vi "Teleop.vi"(10 "Match Info":T1={"Autonomous Elapsed Seconds"=0.0, "TeleOp Elapsed Seconds"=0.0, "Disabled Elapsed Seconds"=0.0, "Visited Autonomous"=FALSE, "Visited TeleOp"=FALSE, "Visited Disabled"=FALSE, "Autonomous Settings"={"Autonomous Style"=enum."Independent", "VI Refnum"=refnum}}, 11 "Call Context":T2) -> ()   [LabVIEW 2019]
doc: "This VI is called for each TeleOp packet received from the DS where the robot is not disabled. It is often used to read from the joysticks and update I/O or to update setpoints for timed control loops. It should complete and return within 20 milliseconds or it may miss DS packets."
uses:
  <vilib>/Rock Robotics/Network Tables/NT Read Boolean.vi
  572ad318-ad2d-41da-8177-273dc494c89e.vi
  <vilib>/Rock Robotics/WPI/ThirdParty/Phoenix-LabVIEW/Motor Controller/Controls/CTRE_Phoenix_MotorControl_ControlMode.ctl
  <vilib>/Rock Robotics/WPI/ThirdParty/Phoenix-LabVIEW/Motor Controller/Controls/CTRE_Phoenix_MotorControl_MotionProfileControlMode.ctl
  <vilib>/Rock Robotics/Network Tables/NT Write Numeric Array.vi
  <vilib>/Rock Robotics/Network Tables/NT Read Number.vi
  <vilib>/Rock Robotics/WPI/DriverStation/WPI_DriverStationDerivedRobotMode.ctl
  <vilib>/Rock Robotics/WPI/DriverStation/WPI_DriverStationMatch Info.ctl
panel:
  out "Btm Mot Prof Count 4":i32
  out "Top Mot Prof Count 4":i32
  out "Mot Prof Active Is Valid 4":bool
  out "Mot Prof Active Is Last 4":bool
  out "Mot Prof  Has Under Run 4":bool
  out "Mot Prof  Is Under Run 4":bool
  out "Mot Prof Active Position 4":dbl
  out "Mot Prof Active Velocity 4":dbl
  out "Btm Mot Prof Count 3":i32
  out "Top Mot Prof Count 3":i32
  out "Mot Prof Active Is Valid 3":bool
  out "Mot Prof Active Is Last 3":bool
  out "Mot Prof  Has Under Run 3":bool
  out "Mot Prof  Is Under Run 3":bool
  out "Mot Prof Active Position 3":dbl
  out "Mot Prof Active Velocity 3":dbl
  out "Btm Mot Prof Count 2":i32
  out "Top Mot Prof Count 2":i32
  out "Mot Prof Active Is Valid 2":bool
  out "Mot Prof Active Is Last 2":bool
  out "Mot Prof  Has Under Run 2":bool
  out "Mot Prof  Is Under Run 2":bool
  out "Mot Prof Active Position 2":dbl
  out "Mot Prof Active Velocity 2":dbl
  out "Is Motion Profile Finished?":bool
  out "Btm Mot Prof Count":i32
  out "Top Mot Prof Count":i32
  out "Mot Prof Active Is Valid":bool
  out "Mot Prof Active Is Last":bool
  out "Mot Prof  Has Under Run":bool
  out "Mot Prof  Is Under Run":bool
  out "Mot Prof Active Position":dbl
  out "Mot Prof Active Velocity":dbl
  out "Sample Slider 0":dbl(slide) scale=0.0..5.0
  out "Sample Boolean 1":bool
  out "Sample Boolean 0":bool
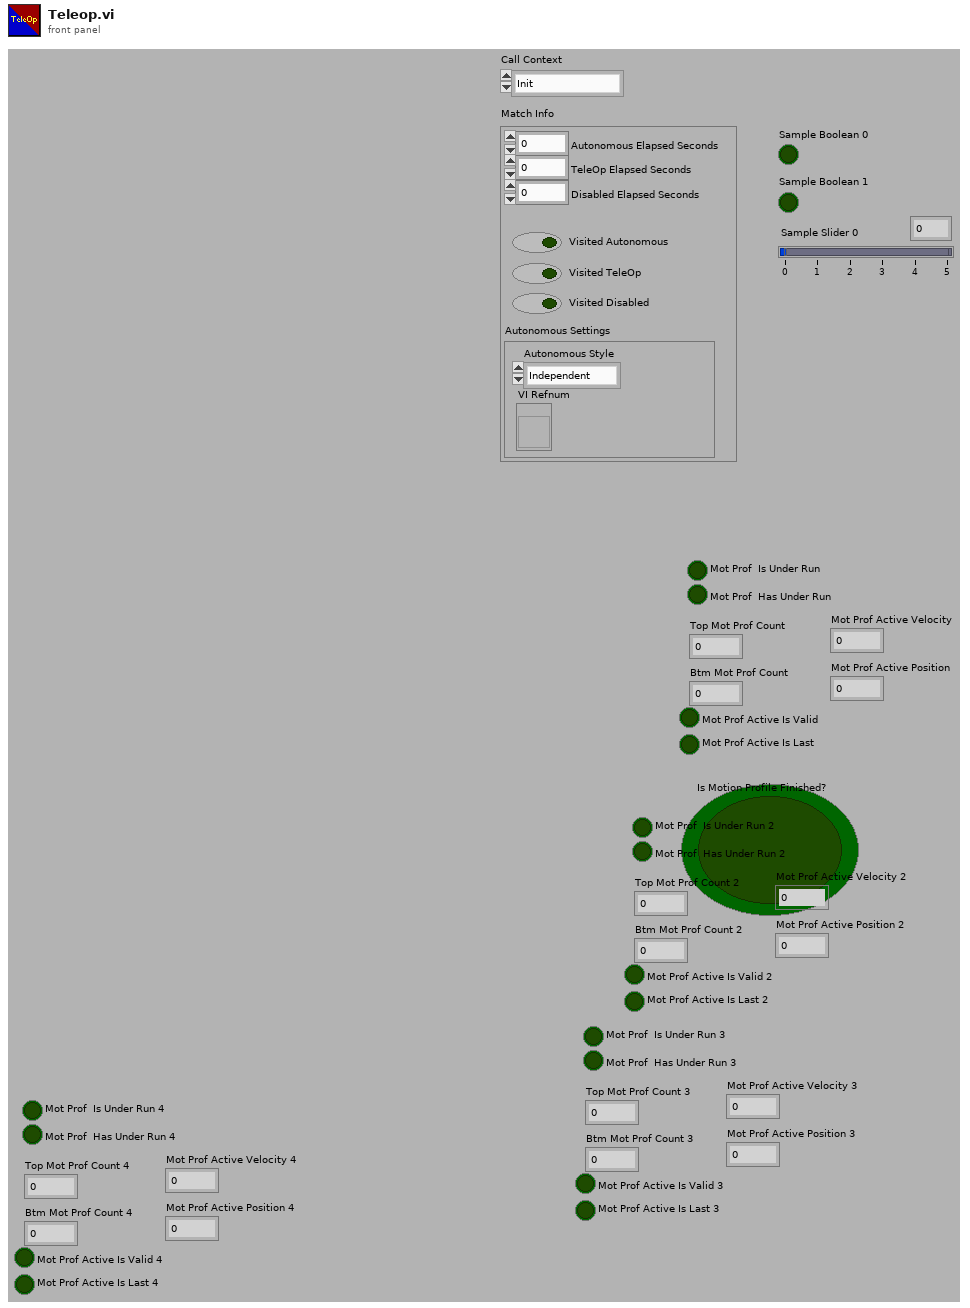
[diagram p1: front panel]
types:
  T1 = typedef "WPI_DriverStationMatch Info.ctl" = cluster{"Autonomous Elapsed Seconds":dbl, "TeleOp Elapsed Seconds":dbl, "Disabled Elapsed Seconds":dbl, "Visited Autonomous":bool, "Visited TeleOp":bool, "Visited Disabled":bool, "Autonomous Settings":cluster{"Autonomous Style":enum16{"Iterative", "Independent"}, "VI Refnum":refnum<vi>}}
  T2 = typedef "WPI_DriverStationDerivedRobotMode.ctl" = enum16{"Init", "Execute", "Stop"}
  T3 = typedef "WPI_MotorControlDeviceRef.ctl" = cluster{"DeviceStatus":errorcluster, "Type":T4, "PWM":cluster{"PWM Channel":T5, "DeadBand":T6}, "CAN":cluster{"Device Number":u8, "SetOutput VI Ref":variant, "GetOutput VI Ref":variant, "Enable VI Ref":variant, "Disable VI Ref":variant, "Data":variant}, "Invert":bool, "DIO PWM":cluster{"PWM \"Enable\" Channel":T5, "DIOChannel":T7, "PWM Rate":dbl}}
  T4 = typedef "WPI_MotorControlType.ctl" = enum16{"PWM", "CAN", "DIO PWM"}
  T5 = typedef "FPGA_DIOPWMChannel.ctl" = enum8{"PWM 0", "PWM 1", "PWM 2", "PWM 3", "PWM 4", "PWM 5", "PWM 6", "PWM 7", "PWM 8", "PWM 9", "PWM MXP 0", "PWM MXP 1", "PWM MXP 2", "PWM MXP 3", "PWM MXP 4", "PWM MXP 5", "PWM MXP 6", "PWM MXP 7", "PWM MXP 8", "PWM MXP 9", "Invalid"}
  T6 = typedef "WPI_PWMDeadband.ctl" = cluster{"Name":string, "maxPositivePwm":i32, "minPositivePwm":i32, "centerPwm":i32, "maxNegativePwm":i32, "minNegativePwm":i32, "angularRange":u16}
  T7 = typedef "FPGA_DIOChannel.ctl" = enum8{"DIO 0", "DIO 1", "DIO 2", "DIO 3", "DIO 4", "DIO 5", "DIO 6", "DIO 7", "DIO 8", "DIO 9", "DIO MXP 0", "DIO MXP 1", "DIO MXP 2", "DIO MXP 3", "DIO MXP 4", "DIO MXP 5", "DIO MXP 6", "DIO MXP 7", "DIO MXP 8", "DIO MXP 9", "DIO MXP 10", "DIO MXP 11", "DIO MXP 12", "DIO MXP 13", "DIO MXP 14", "DIO MXP 15", "SPI Port CS1", "SPI Port CS2", "SPI Port CS3", "SPI Port MISO", "SPI Port MOSI", "Invalid"}
  T8 = typedef "WPI_RobotDriveDevRef.ctl" = cluster{"DevStatus":errorcluster, "Motors[]":T3[], "Square Inputs":bool, "Max Output":dbl}
  T9 = typedef "WPI_JoystickDevRef.ctl" = cluster{"Device":T10}
  T10 = typedef "WPI_JoystickDeviceEnum.ctl" = enum16{"USB 0", "USB 1", "USB 2", "USB 3", "USB 4", "USB 5"}
  T11 = cluster{"Top Buffer Remaining":i32, "Top Buffer Count":i32, "Bottom Buffer Count":i32, "Has Underrun?":bool, "Is Underrun?":bool, "Active Point Valid?":bool, "Is Last?":bool, "Profile Slot Select 0":i32, "Output Enable":i32, "Time Duration (ms)":i32, "Profile Slot Select 1":i32}
  T12 = typedef "CTRE_Phoenix_MotorControl_ControlMode.ctl" = u16
  T13 = typedef "CTRE_Phoenix_MotorControl_MotionProfileControlMode.ctl" = u16
  T14 = typedef "CTRE_Phoenix_MotorControl_BufferedTrajectoryPointStream_DeviceRef.ctl" = cluster{"Handle":u64, "Library Path":path}
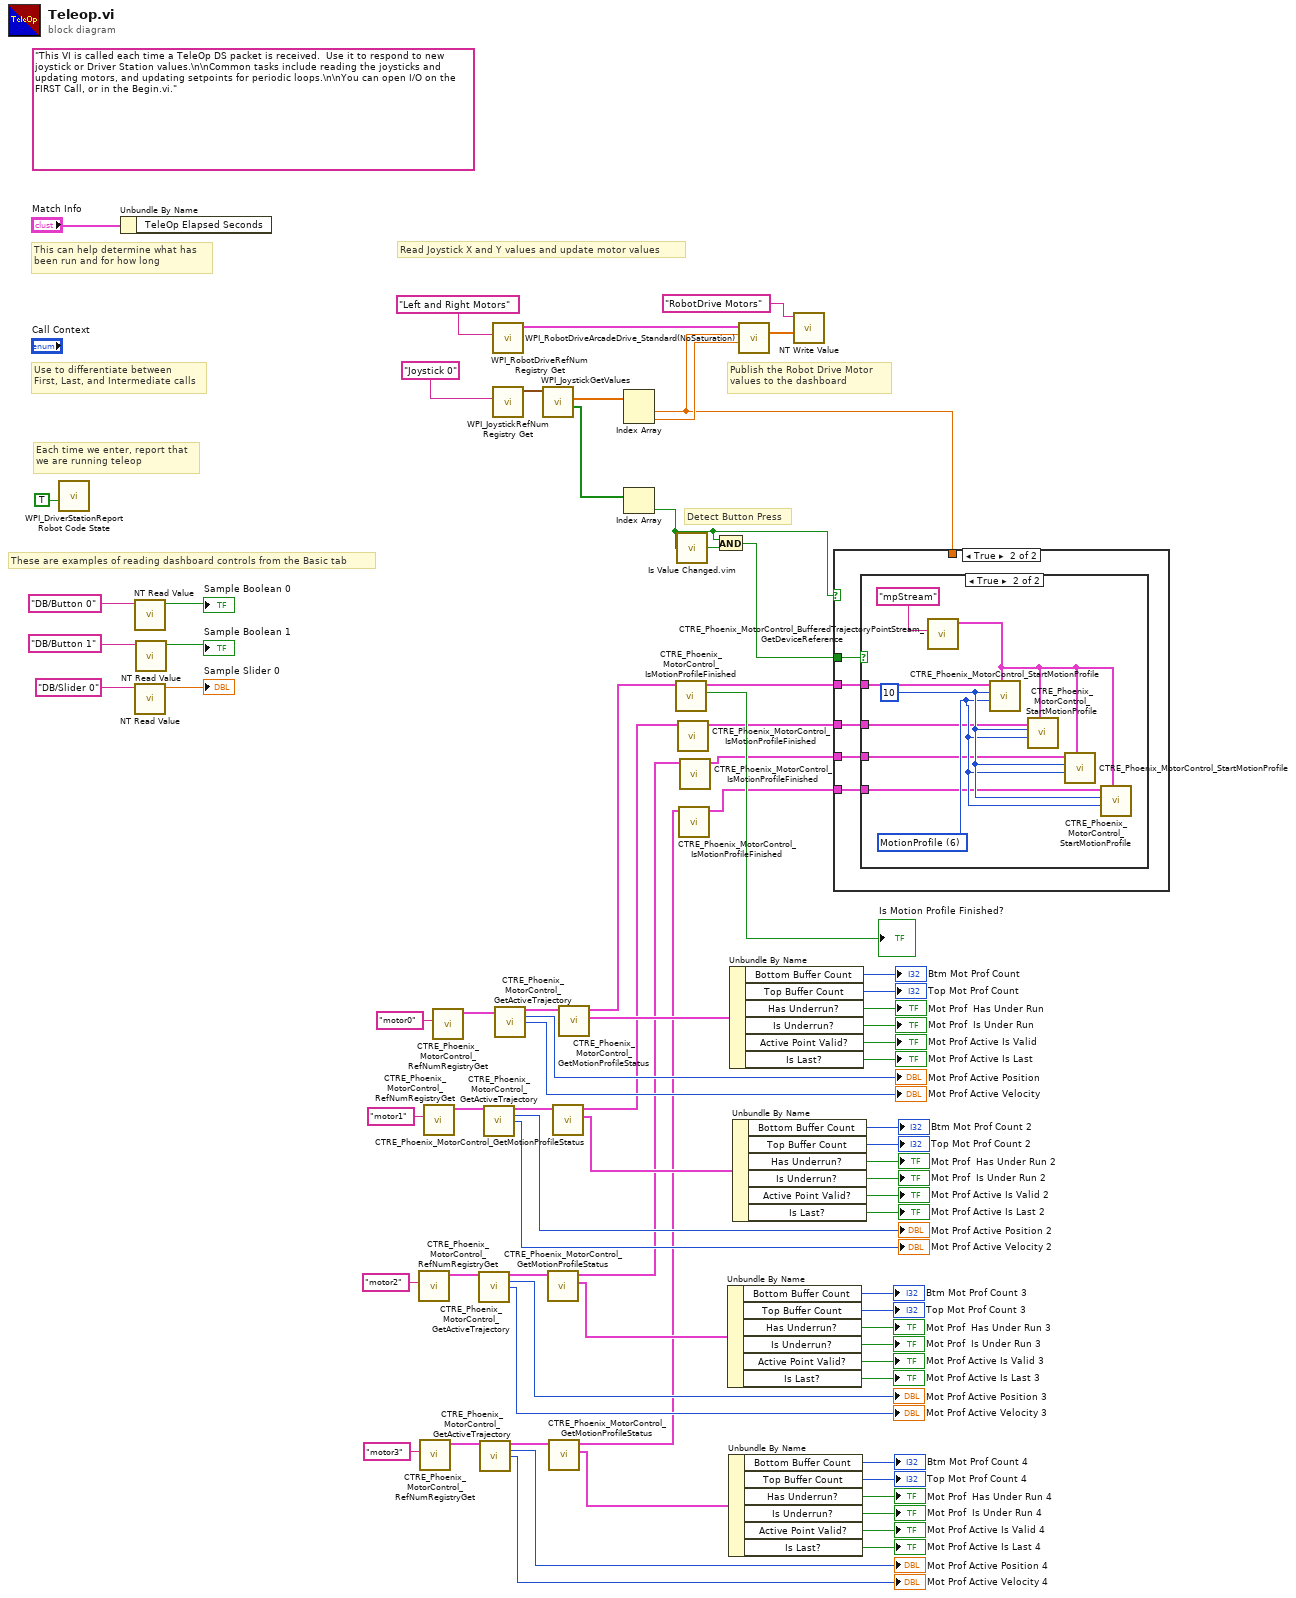
[diagram p0: block diagram]
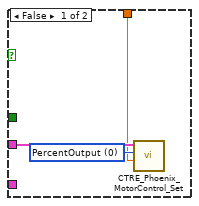
[diagram p2: hidden frame]
diagram:
  (unwired) "This VI is called each time a TeleOp DS packet is received.  Use it to respond to new joystick or Driver Station values.\n\nCommon tasks include reading the joysticks and updating motors, and updating setpoints for periodic loops.\n\nYou can open I/O on the FIRST Call, or in the Begin.vi."
  # "Detect Button Press"
  # "These are examples of reading dashboard controls from the Basic tab"
  # "Publish the Robot Drive Motor\nvalues to the dashboard"
  # "Each time we enter, report that\nwe are running teleop"
  # "Use to differentiate between\nFirst, Last, and Intermediate calls"
  # "This can help determine what has\nbeen run and for how long"
  # "Read Joystick X and Y values and update motor values"
  n1 = call <vilib>:"WPI_DriverStationReport Robot Code State.vi"("TeleOp"=TRUE ("Autonomous")) -> ()  [unwired: 10 in, 1 out]
  n2 = Unbundle By Name("Match Info") -> ()  [unwired: 1 out]
  n3 = call-poly <vilib>:"NT Read Value.vi"("Name"="DB/Button 0" ("refnum name")) -> ("Boolean"=→"Sample Boolean 0":bool)  [unwired: 9 in, 1 out]
  n4 = call-poly <vilib>:"NT Read Value.vi"("Name"="DB/Slider 0" ("refnum name")) -> ("Numeric"=→"Sample Slider 0":dbl)  [unwired: 9 in, 1 out]
  n5 = call-poly <vilib>:"NT Read Value.vi"("Name"="DB/Button 1" ("refnum name")) -> ("Boolean"=→"Sample Boolean 1":bool)  [unwired: 9 in, 1 out]
  n6 = call <vilib>:"CTRE_Phoenix_MotorControl_RefNumRegistryGet.vi"("refnum name"="motor2") -> ("PhoenixMotorControlDevRef"=w6:T3)  [unwired: 9 in, 1 out]
  n7 = call <vilib>:"CTRE_Phoenix_MotorControl_RefNumRegistryGet.vi"("refnum name"="motor3") -> ("PhoenixMotorControlDevRef"=w4:T3)  [unwired: 9 in, 1 out]
  n8 = call <vilib>:"CTRE_Phoenix_MotorControl_RefNumRegistryGet.vi"("refnum name"="motor1") -> ("PhoenixMotorControlDevRef"=w41:T3)  [unwired: 9 in, 1 out]
  n9 = call <vilib>:"CTRE_Phoenix_MotorControl_RefNumRegistryGet.vi"("refnum name"="motor0") -> ("PhoenixMotorControlDevRef"=w44:T3)  [unwired: 9 in, 1 out]
  n10 = call <vilib>:"CTRE_Phoenix_MotorControl_GetActiveTrajectory.vi"("PhoenixMotorControlDevRef"=w6) -> ("PhoenixMotorControlDevRef"=w1:T3, "Position (Sensor Units)"=→"Mot Prof Active Position 3":i32, "Velocity (Sensor Units per 100 ms)"=→"Mot Prof Active Velocity 3":i32)  [unwired: 10 in, 2 out]
  n11 = call <vilib>:"CTRE_Phoenix_MotorControl_GetActiveTrajectory.vi"("PhoenixMotorControlDevRef"=w4) -> ("PhoenixMotorControlDevRef"=w2:T3, "Position (Sensor Units)"=→"Mot Prof Active Position 4":i32, "Velocity (Sensor Units per 100 ms)"=→"Mot Prof Active Velocity 4":i32)  [unwired: 10 in, 2 out]
  n12 = call <vilib>:"CTRE_Phoenix_MotorControl_GetActiveTrajectory.vi"("PhoenixMotorControlDevRef"=w41) -> ("PhoenixMotorControlDevRef"=w37:T3, "Position (Sensor Units)"=→"Mot Prof Active Position 2":i32, "Velocity (Sensor Units per 100 ms)"=→"Mot Prof Active Velocity 2":i32)  [unwired: 10 in, 2 out]
  n13 = call <vilib>:"WPI_RobotDriveRefNum Registry Get.vi"("refnum name"="Left and Right Motors") -> ("RobotDriveDevRef"=w76:T8)  [unwired: 1 in, 9 out]
  n14 = call <vilib>:"WPI_JoystickRefNum Registry Get.vi"("refnum name"="Joystick 0") -> ("JoystickDevRef"=w74:T9)  [unwired: 1 in, 9 out]
  n15 = call <vilib>:"CTRE_Phoenix_MotorControl_GetActiveTrajectory.vi"("PhoenixMotorControlDevRef"=w44) -> ("PhoenixMotorControlDevRef"=w51:T3, "Position (Sensor Units)"=→"Mot Prof Active Position":i32, "Velocity (Sensor Units per 100 ms)"=→"Mot Prof Active Velocity":i32)  [unwired: 10 in, 2 out]
  n16 = call <vilib>:"WPI_JoystickGetValues.vi"("JoystickDevRef"=w74) -> ("Buttons"=w62:bool[], "Axes"=w71:dbl[])  [unwired: 6 in, 3 out]
  n17 = call <vilib>:"CTRE_Phoenix_MotorControl_GetMotionProfileStatus.vi"("PhoenixMotorControlDevRef"=w1) -> ("Motion Profile Status"=w19:T11, "PhoenixMotorControlDevRef"=w5:T3)  [unwired: 8 in, 1 out]
  n18 = call <vilib>:"CTRE_Phoenix_MotorControl_GetMotionProfileStatus.vi"("PhoenixMotorControlDevRef"=w2) -> ("Motion Profile Status"=w9:T11, "PhoenixMotorControlDevRef"=w3:T3)  [unwired: 8 in, 1 out]
  n19 = call <vilib>:"CTRE_Phoenix_MotorControl_GetMotionProfileStatus.vi"("PhoenixMotorControlDevRef"=w37) -> ("Motion Profile Status"=w29:T11, "PhoenixMotorControlDevRef"=w36:T3)  [unwired: 8 in, 1 out]
  n20 = call <vilib>:"CTRE_Phoenix_MotorControl_GetMotionProfileStatus.vi"("PhoenixMotorControlDevRef"=w51) -> ("Motion Profile Status"=w58:T11, "PhoenixMotorControlDevRef"=w50:T3)  [unwired: 8 in, 1 out]
  n21 = Index Array(array=w71) -> (element #1=w45:dbl, element #2=w72:dbl)  [unwired: 2 in]
  n22 = Index Array(array=w62) -> (element=w46:bool)  [unwired: 1 in]
  n23 = call <vilib>:"CTRE_Phoenix_MotorControl_IsMotionProfileFinished.vi"("PhoenixMotorControlDevRef"=w50) -> ("Is Motion Profile Finished?"=→"Is Motion Profile Finished?":bool, "PhoenixMotorControlDevRef"=w49:T3)  [unwired: 8 in, 1 out]
  n24 = call "Is Value Changed.vim"("value"=w46) -> ("changed or first call?"=w61:bool)
  n25 = call <vilib>:"CTRE_Phoenix_MotorControl_IsMotionProfileFinished.vi"("PhoenixMotorControlDevRef"=w36) -> ("PhoenixMotorControlDevRef"=w40:T3)  [unwired: 8 in, 2 out]
  n26 = call <vilib>:"CTRE_Phoenix_MotorControl_IsMotionProfileFinished.vi"("PhoenixMotorControlDevRef"=w3) -> ("PhoenixMotorControlDevRef"=w38:T3)  [unwired: 8 in, 2 out]
  n27 = call <vilib>:"CTRE_Phoenix_MotorControl_IsMotionProfileFinished.vi"("PhoenixMotorControlDevRef"=w5) -> ("PhoenixMotorControlDevRef"=w39:T3)  [unwired: 8 in, 2 out]
  n28 = And(x=w46, y=w61) -> (x .and. y?=w47:bool)
  n29 = Unbundle By Name(w19) -> ("Bottom Buffer Count"=→"Btm Mot Prof Count 3":i32, "Top Buffer Count"=→"Top Mot Prof Count 3":i32, "Has Underrun?"=→"Mot Prof  Has Under Run 3":bool, "Is Underrun?"=→"Mot Prof  Is Under Run 3":bool, "Active Point Valid?"=→"Mot Prof Active Is Valid 3":bool, "Is Last?"=→"Mot Prof Active Is Last 3":bool)
  n30 = Unbundle By Name(w9) -> ("Bottom Buffer Count"=→"Btm Mot Prof Count 4":i32, "Top Buffer Count"=→"Top Mot Prof Count 4":i32, "Has Underrun?"=→"Mot Prof  Has Under Run 4":bool, "Is Underrun?"=→"Mot Prof  Is Under Run 4":bool, "Active Point Valid?"=→"Mot Prof Active Is Valid 4":bool, "Is Last?"=→"Mot Prof Active Is Last 4":bool)
  n31 = Unbundle By Name(w58) -> ("Bottom Buffer Count"=→"Btm Mot Prof Count":i32, "Top Buffer Count"=→"Top Mot Prof Count":i32, "Has Underrun?"=→"Mot Prof  Has Under Run":bool, "Is Underrun?"=→"Mot Prof  Is Under Run":bool, "Active Point Valid?"=→"Mot Prof Active Is Valid":bool, "Is Last?"=→"Mot Prof Active Is Last":bool)
  n32 = Unbundle By Name(w29) -> ("Bottom Buffer Count"=→"Btm Mot Prof Count 2":i32, "Top Buffer Count"=→"Top Mot Prof Count 2":i32, "Has Underrun?"=→"Mot Prof  Has Under Run 2":bool, "Is Underrun?"=→"Mot Prof  Is Under Run 2":bool, "Active Point Valid?"=→"Mot Prof Active Is Valid 2":bool, "Is Last?"=→"Mot Prof Active Is Last 2":bool)
  n33 = call <vilib>:"WPI_RobotDriveArcadeDrive_Standard(NoSaturation).vi"("Y axis value"=w72, "X axis value"=w45, "RobotDriveDevRef"=w76) -> ("Motor Values"=w64:dbl[])  [unwired: 1 in, 7 out]
  n34 = call-poly <vilib>:"NT Write Value.vi"("Numeric Array"=w64, "Name"="RobotDrive Motors") -> ()  [unwired: 9 in, 1 out]
  n35 = case shown="True" w46 {
    tunnel: w49 -> [w81 w86]
    tunnel: w47 -> [_ w85]
    tunnel: w45 -> [w79 _]
    tunnel: w40 -> [_ w84]
    tunnel: w39 -> [_ w83]
    tunnel: w38 -> [_ w82]
    frame False {
      w80 = T12 0 items=["PercentOutput"=0, "Position"=1, "Velocity"=2, "Current"=3, "Follower"=5, "MotionProfile"=6, "MotionMagic"=7, "MotionProfileArc"=10, "Disabled"=15] ("Control Mode")
      n36 = call <vilib>:"CTRE_Phoenix_MotorControl_Set.vi"("Output"=w79, "Control Mode"=w80, "PhoenixMotorControlDevRef"=w81) -> ()  [unwired: 7 in, 2 out]
    }
    frame True {
      n37 = case shown="True" w85 {
        tunnel: w86 -> [_ w90]
        tunnel: w84 -> [_ w89]
        tunnel: w83 -> [_ w88]
        tunnel: w82 -> [_ w87]
        frame False {
        }
        frame True {
          w93 = u32 10 ("minBufferedPts")
          w92 = T13 6 items=["MotionProfile"=6, "MotionProfileArc"=10] ("Control Mode")
          n38 = call <vilib>:"CTRE_Phoenix_MotorControl_BufferedTrajectoryPointStream_GetDeviceReference.vi"("refnum name"="mpStream") -> ("BufferedTrajectoryPointStream_DevRef"=w91:T14)  [unwired: 9 in, 1 out]
          n39 = call <vilib>:"CTRE_Phoenix_MotorControl_StartMotionProfile.vi"("BufferedTrajectoryPointStream_DevRef"=w91, "Control Mode"=w92, "minBufferedPts"=w93, "PhoenixMotorControlDevRef"=w90) -> ()  [unwired: 6 in, 2 out]
          n40 = call <vilib>:"CTRE_Phoenix_MotorControl_StartMotionProfile.vi"("BufferedTrajectoryPointStream_DevRef"=w91, "Control Mode"=w92, "minBufferedPts"=w93, "PhoenixMotorControlDevRef"=w89) -> ()  [unwired: 6 in, 2 out]
          n41 = call <vilib>:"CTRE_Phoenix_MotorControl_StartMotionProfile.vi"("BufferedTrajectoryPointStream_DevRef"=w91, "Control Mode"=w92, "minBufferedPts"=w93, "PhoenixMotorControlDevRef"=w88) -> ()  [unwired: 6 in, 2 out]
          n42 = call <vilib>:"CTRE_Phoenix_MotorControl_StartMotionProfile.vi"("BufferedTrajectoryPointStream_DevRef"=w91, "Control Mode"=w92, "minBufferedPts"=w93, "PhoenixMotorControlDevRef"=w87) -> ()  [unwired: 6 in, 2 out]
        }
      }
    }
  }
